vi "get piece from line 2.vi"   [LabVIEW 2018]
types:
  T1 = enum16{"shoulder", "elbow", "wrist", "base", "gripper"}
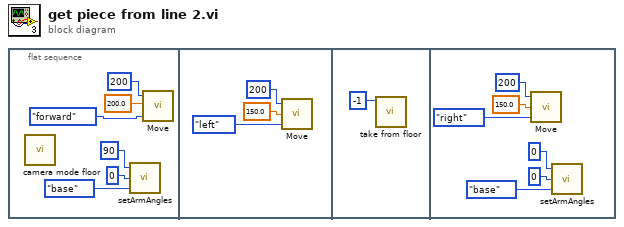
[diagram p0: block diagram]
diagram:
  n1 = flat-sequence {
    frame #0 {
      n2 = call "camera mode floor.vi"() -> ()  [unwired: 12 in]
      n3 = call "setArmAngles.vi"("Enum"=T1."base", "speed"=0, "angle"=90) -> ()  [unwired: 1 in]
      n4 = call "Move.vi"("Enum"=enum16{"forward", "backward", "left", "right"}."forward", "distance"=200.0, "speed"=200) -> ()  [unwired: 1 in]
    }
    frame #1 {
      n5 = call "Move.vi"("Enum"=enum16{"forward", "backward", "left", "right"}."left", "distance"=150.0, "speed"=200) -> ()  [unwired: 1 in]
    }
    frame #2 {
      n6 = call "take from floor.vi"("m"=-1) -> ()  [unwired: 11 in]
    }
    frame #3 {
      n7 = call "Move.vi"("Enum"=enum16{"forward", "backward", "left", "right"}."right", "distance"=150.0, "speed"=200) -> ()  [unwired: 1 in]
      n8 = call "setArmAngles.vi"("Enum"=T1."base", "speed"=0, "angle"=0) -> ()  [unwired: 1 in]
    }
  }
